vi "Configure Active Trace.vi"(8 "error in (no error)":errorcluster, 10 "Active Trace Number (1)":u16=1 min=1, 11 "SA-ESA in":refnum<class "SA-ESA.lvclass">) -> (0 "error out":errorcluster, 3 "SA-ESA out":refnum<class "SA-ESA.lvclass">)   [LabVIEW 2020, in "SA-ESA.lvclass"]
uses:
  SA-ESA.lvclass
  C:/Sandbox/Git_Sandbox/WiSpry Test Framework source code (LV20)/WiSpry Test Framework/Instruments/Spectrum Analyzer/Spectrum Analyzer.lvclass
  Spectrum Analyzer.lvclass/Spectrum Analyzer.ctl
  Spectrum Analyzer.lvclass
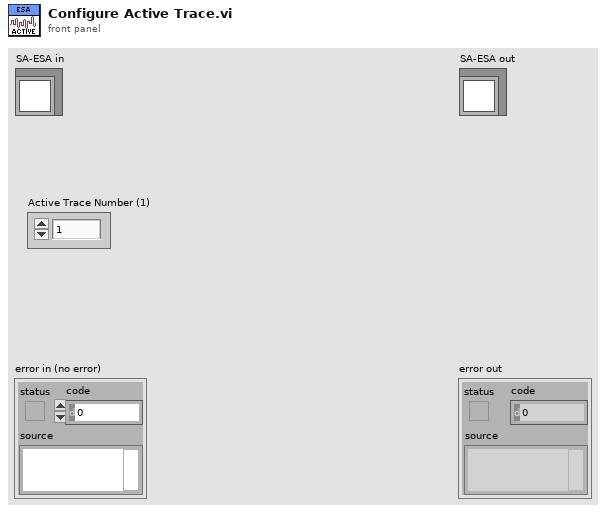
[diagram p1: front panel]
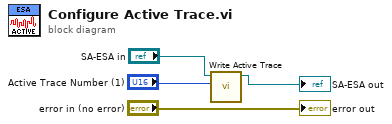
[diagram p0: block diagram]
diagram:
  n1 = call "Write Active Trace.vi"("Active Trace"="Active Trace Number (1)", "Spectrum Analyzer in"="SA-ESA in") -> ("Spectrum Analyzer out"=→"SA-ESA out":refnum<class "SA-ESA.lvclass">)  [unwired: 9 in]
  "error out" <- "error in (no error)"
